vi "arduino.vi"   [LabVIEW 2016]
uses:
  <vilib>/LabVIEW Interface for Arduino/LabVIEW Interface for Arduino.lvlib
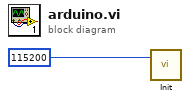
[diagram p0: block diagram]
diagram:
  n1 = call <vilib>:"Init.vi"("Baud Rate (115200)"=u32 115200) -> ()  [unwired: 17 in, 2 out]
